vi "rsidr_core_global.vi"() -> ()   [LabVIEW 2020, in "Rohde&Schwarz CMWXP NR FR1 Measurement.lvlib"] (continued)
"Access"=enum."Read Only", "Range Table"="", "Read Callback"="", "Write Callback"="", "Range Callback"="", "Check Callback"="", "Rngtable Callback"="", "Coerce Callback"="", "Supported Models"="", "Instrument Options"="", "Check Status Callback"="", "Flags"=0, "Help"="Returns the values of the power dynamics traces. Each value is sampled with 48 Ts, corresponding to 1.5625 us. The results of the maximum traces can be retrieved.\n\nAvailable Repeated Capabilities:\ninstance: i0, i1, i2, i3, i4, i5, i6, i7, i8, i9, i10, i11, i12, i13, i14, i15, i16, i17, i18, i19, i20, i21, i22, i23, i24, i25, i26, i27, i28, i29, i30, i31, i32\r\n\nRemote-control command(s):\nFETCh:NRSub:MEAS<i>:PRACh:TRACe:PDYNamics:MAXimum?"}, {"Level"=3, "Class Only"=TRUE, "Identifier"="", "Descriptive Name"="Modulation", "Data Type"=enum."ViInt32", "Command"="", "Access"=enum."Read Only", "Range Table"="", "Read Callback"="", "Write Callback"="", "Range Callback"="", "Check Callback"="", "Rngtable Callback"="", "Coerce Callback"="", "Supported Models"="", "Instrument Options"="", "Check Status Callback"="", "Flags"=0, "Help"="The following commands return the statistical modulation results."}, {"Level"=4, "Class Only"=FALSE, "Identifier"="RSCMWXPNRFR1M_ATTR_QUERY_PRACH_MODULATION_CURRENT_LIMIT_CHECK_RESULTS", "Descriptive Name"="Query PRACH Modulation Current Limit Check Results", "Data Type"=enum."RawString", "Command"="CALC:NRS:MEAS{instance}:PRAC:MOD:CURR?", "Access"=enum."Read Only", "Range Table"="", "Read Callback"="", "Write Callback"="", "Range Callback"="", "Check Callback"="", "Rngtable Callback"="", "Coerce Callback"="", "Supported Models"="", "Instrument Options"="", "Check Status Callback"="", "Flags"=0, "Help"="Returns the limit check results for the current single value results.\n\nAvailable Repeated Capabilities:\ninstance: i0, i1, i2, i3, i4, i5, i6, i7, i8, i9, i10, i11, i12, i13, i14, i15, i16, i17, i18, i19, i20, i21, i22, i23, i24, i25, i26, i27, i28, i29, i30, i31, i32\r\n\nRemote-control command(s):\nCALCulate:NRSub:MEAS<i>:PRACh:MODulation:CURRent?"}, {"Level"=4, "Class Only"=FALSE, "Identifier"="RSCMWXPNRFR1M_ATTR_QUERY_PRACH_MODULATION_AVERAGE_LIMIT_CHECK_RESULTS", "Descriptive Name"="Query PRACH Modulation Average Limit Check Results", "Data Type"=enum."RawString", "Command"="CALC:NRS:MEAS{instance}:PRAC:MOD:AVER?", "Access"=enum."Read Only", "Range Table"="", "Read Callback"="", "Write Callback"="", "Range Callback"="", "Check Callback"="", "Rngtable Callback"="", "Coerce Callback"="", "Supported Models"="", "Instrument Options"="", "Check Status Callback"="", "Flags"=0, "Help"="Returns the limit check results for the average single value results.\n\nAvailable Repeated Capabilities:\ninstance: i0, i1, i2, i3, i4, i5, i6, i7, i8, i9, i10, i11, i12, i13, i14, i15, i16, i17, i18, i19, i20, i21, i22, i23, i24, i25, i26, i27, i28, i29, i30, i31, i32\r\n\nRemote-control command(s):\nCALCulate:NRSub:MEAS<i>:PRACh:MODulation:AVERage?"}, {"Level"=4, "Class Only"=FALSE, "Identifier"="RSCMWXPNRFR1M_ATTR_READ_PRACH_MODULATION_CURRENT_RESULTS", "Descriptive Name"="Read PRACH Modulation Current Results", "Data Type"=enum."RawString", "Command"="READ:NRS:MEAS{instance}:PRAC:MOD:CURR?", "Access"=enum."Read Only", "Range Table"="", "Read Callback"="", "Write Callback"="", "Range Callback"="", "Check Callback"="", "Rngtable Callback"="", "Coerce Callback"="", "Supported Models"="", "Instrument Options"="", "Check Status Callback"="", "Flags"=0, "Help"="Starts a new single shot measurement and returns the current single value results.\n\nAvailable Repeated Capabilities:\ninstance: i0, i1, i2, i3, i4, i5, i6, i7, i8, i9, i10, i11, i12, i13, i14, i15, i16, i17, i18, i19, i20, i21, i22, i23, i24, i25, i26, i27, i28, i29, i30, i31, i32\r\n\nRemote-control command(s):\nREAD:NRSub:MEAS<i>:PRACh:MODulation:CURRent?"}, {"Level"=4, "Class Only"=FALSE, "Identifier"="RSCMWXPNRFR1M_ATTR_READ_PRACH_MODULATION_AVERAGE_RESULTS", "Descriptive Name"="Read PRACH Modulation Average Results", "Data Type"=enum."RawString", "Command"="READ:NRS:MEAS{instance}:PRAC:MOD:AVER?", "Access"=enum."Read Only", "Range Table"="", "Read Callback"="", "Write Callback"="", "Range Callback"="", "Check Callback"="", "Rngtable Callback"="", "Coerce Callback"="", "Supported Models"="", "Instrument Options"="", "Check Status Callback"="", "Flags"=0, "Help"="Starts a new single shot measurement and returns the average single value results.\n\nAvailable Repeated Capabilities:\ninstance: i0, i1, i2, i3, i4, i5, i6, i7, i8, i9, i10, i11, i12, i13, i14, i15, i16, i17, i18, i19, i20, i21, i22, i23, i24, i25, i26, i27, i28, i29, i30, i31, i32\r\n\nRemote-control command(s):\nREAD:NRSub:MEAS<i>:PRACh:MODulation:AVERage?"}, {"Level"=4, "Class Only"=FALSE, "Identifier"="RSCMWXPNRFR1M_ATTR_READ_PRACH_MODULATION_STANDARD_DEVIATION_RESULTS", "Descriptive Name"="Read PRACH Modulation Standard Deviation Results", "Data Type"=enum."RawString", "Command"="READ:NRS:MEAS{instance}:PRAC:MOD:SDEV?", "Access"=enum."Read Only", "Range Table"="", "Read Callback"="", "Write Callback"="", "Range Callback"="", "Check Callback"="", "Rngtable Callback"="", "Coerce Callback"="", "Supported Models"="", "Instrument Options"="", "Check Status Callback"="", "Flags"=0, "Help"="Starts a new single shot measurement and returns the standard deviation single value results.\n\nAvailable Repeated Capabilities:\ninstance: i0, i1, i2, i3, i4, i5, i6, i7, i8, i9, i10, i11, i12, i13, i14, i15, i16, i17, i18, i19, i20, i21, i22, i23, i24, i25, i26, i27, i28, i29, i30, i31, i32\r\n\nRemote-control command(s):\nREAD:NRSub:MEAS<i>:PRACh:MODulation:SDEViation?"}, {"Level"=4, "Class Only"=FALSE, "Identifier"="RSCMWXPNRFR1M_ATTR_FETCH_PRACH_MODULATION_CURRENT_RESULTS", "Descriptive Name"="Fetch PRACH Modulation Current Results", "Data Type"=enum."RawString", "Command"="FETC:NRS:MEAS{instance}:PRAC:MOD:CURR?", "Access"=enum."Read Only", "Range Table"="", "Read Callback"="", "Write Callback"="", "Range Callback"="", "Check Callback"="", "Rngtable Callback"="", "Coerce Callback"="", "Supported Models"="", "Instrument Options"="", "Check Status Callback"="", "Flags"=0, "Help"="Returns the current single value results.\n\nAvailable Repeated Capabilities:\ninstance: i0, i1, i2, i3, i4, i5, i6, i7, i8, i9, i10, i11, i12, i13, i14, i15, i16, i17, i18, i19, i20, i21, i22, i23, i24, i25, i26, i27, i28, i29, i30, i31, i32\r\n\nRemote-control command(s):\nFETCh:NRSub:MEAS<i>:PRACh:MODulation:CURRent?"}, {"Level"=4, "Class Only"=FALSE, "Identifier"="RSCMWXPNRFR1M_ATTR_FETCH_PRACH_MODULATION_AVERAGE_RESULTS", "Descriptive Name"="Fetch PRACH Modulation Average Results", "Data Type"=enum."RawString", "Command"="FETC:NRS:MEAS{instance}:PRAC:MOD:AVER?", "Access"=enum."Read Only", "Range Table"="", "Read Callback"="", "Write Callback"="", "Range Callback"="", "Check Callback"="", "Rngtable Callback"="", "Coerce Callback"="", "Supported Models"="", "Instrument Options"="", "Check Status Callback"="", "Flags"=0, "Help"="Returns the average single value results.\n\nAvailable Repeated Capabilities:\ninstance: i0, i1, i2, i3, i4, i5, i6, i7, i8, i9, i10, i11, i12, i13, i14, i15, i16, i17, i18, i19, i20, i21, i22, i23, i24, i25, i26, i27, i28, i29, i30, i31, i32\r\n\nRemote-control command(s):\nFETCh:NRSub:MEAS<i>:PRACh:MODulation:AVERage?"}, {"Level"=4, "Class Only"=FALSE, "Identifier"="RSCMWXPNRFR1M_ATTR_FETCH_PRACH_MODULATION_STANDARD_DEVIATION_RESULTS", "Descriptive Name"="Fetch PRACH Modulation Standard Deviation Results", "Data Type"=enum."RawString", "Command"="FETC:NRS:MEAS{instance}:PRAC:MOD:SDEV?", "Access"=enum."Read Only", "Range Table"="", "Read Callback"="", "Write Callback"="", "Range Callback"="", "Check Callback"="", "Rngtable Callback"="", "Coerce Callback"="", "Supported Models"="", "Instrument Options"="", "Check Status Callback"="", "Flags"=0, "Help"="Returns the standard deviation single value results.\n\nAvailable Repeated Capabilities:\ninstance: i0, i1, i2, i3, i4, i5, i6, i7, i8, i9, i10, i11, i12, i13, i14, i15, i16, i17, i18, i19, i20, i21, i22, i23, i24, i25, i26, i27, i28, i29, i30, i31, i32\r\n\nRemote-control command(s):\nFETCh:NRSub:MEAS<i>:PRACh:MODulation:SDEViation?"}, {"Level"=4, "Class Only"=FALSE, "Identifier"="RSCMWXPNRFR1M_ATTR_QUERY_PRACH_MODULATION_EXTREME_LIMIT_CHECK_RESULTS", "Descriptive Name"="Query PRACH Modulation Extreme Limit Check Results", "Data Type"=enum."RawString", "Command"="CALC:NRS:MEAS{instance}:PRAC:MOD:EXTR?", "Access"=enum."Read Only", "Range Table"="", "Read Callback"="", "Write Callback"="", "Range Callback"="", "Check Callback"="", "Rngtable Callback"="", "Coerce Callback"="", "Supported Models"="", "Instrument Options"="", "Check Status Callback"="", "Flags"=0, "Help"="Returns the limit check results for modulation extreme values.\n\nAvailable Repeated Capabilities:\ninstance: i0, i1, i2, i3, i4, i5, i6, i7, i8, i9, i10, i11, i12, i13, i14, i15, i16, i17, i18, i19, i20, i21, i22, i23, i24, i25, i26, i27, i28, i29, i30, i31, i32\r\n\nRemote-control command(s):\nCALCulate:NRSub:MEAS<i>:PRACh:MODulation:EXTReme?"}, {"Level"=4, "Class Only"=FALSE, "Identifier"="RSCMWXPNRFR1M_ATTR_READ_PRACH_MODULATION_EXTREME_RESULTS", "Descriptive Name"="Read PRACH Modulation Extreme Results", "Data Type"=enum."RawString", "Command"="READ:NRS:MEAS{instance}:PRAC:MOD:EXTR?", "Access"=enum."Read Only", "Range Table"="", "Read Callback"="", "Write Callback"="", "Range Callback"="", "Check Callback"="", "Rngtable Callback"="", "Coerce Callback"="", "Supported Models"="", "Instrument Options"="", "Check Status Callback"="", "Flags"=0, "Help"="Starts a new single shot measurement and returns the extreme single value results.\n\nAvailable Repeated Capabilities:\ninstance: i0, i1, i2, i3, i4, i5, i6, i7, i8, i9, i10, i11, i12, i13, i14, i15, i16, i17, i18, i19, i20, i21, i22, i23, i24, i25, i26, i27, i28, i29, i30, i31, i32\r\n\nRemote-control command(s):\nREAD:NRSub:MEAS<i>:PRACh:MODulation:EXTReme?"}, {"Level"=4, "Class Only"=FALSE, "Identifier"="RSCMWXPNRFR1M_ATTR_FETCH_PRACH_MODULATION_EXTREME_RESULTS", "Descriptive Name"="Fetch PRACH Modulation Extreme Results", "Data Type"=enum."RawString", "Command"="FETC:NRS:MEAS{instance}:PRAC:MOD:EXTR?", "Access"=enum."Read Only", "Range Table"="", "Read Callback"="", "Write Callback"="", "Range Callback"="", "Check Callback"="", "Rngtable Callback"="", "Coerce Callback"="", "Supported Models"="", "Instrument Options"="", "Check Status Callback"="", "Flags"=0, "Help"="Returns the extreme single value results.\n\nAvailable Repeated Capabilities:\ninstance: i0, i1, i2, i3, i4, i5, i6, i7, i8, i9, i10, i11, i12, i13, i14, i15, i16, i17, i18, i19, i20, i21, i22, i23, i24, i25, i26, i27, i28, i29, i30, i31, i32\r\n\nRemote-control command(s):\nFETCh:NRSub:MEAS<i>:PRACh:MODulation:EXTReme?"}, {"Level"=4, "Class Only"=FALSE, "Identifier"="RSCMWXPNRFR1M_ATTR_READ_PRACH_MODULATION_EVM_POWER_VS_PREAMBLE_RESULTS", "Descriptive Name"="Read PRACH Modulation EVM / Power Vs Preamble Results", "Data Type"=enum."RawString", "Command"="READ:NRS:MEAS{instance}:PRAC:MOD:PRE{preamble}?", "Access"=enum."Read Only", "Range Table"="", "Read Callback"="", "Write Callback"="", "Range Callback"="", "Check Callback"="", "Rngtable Callback"="", "Coerce Callback"="", "Supported Models"="", "Instrument Options"="", "Check Status Callback"="", "Flags"=0, "Help"="Starts a new single shot measurement and returns the single value results of the 'EVM vs Preamble' and 'Power vs Preamble' squares, for a selected preamble.\n\nAvailable Repeated Capabilities:\ninstance: i0, i1, i2, i3, i4, i5, i6, i7, i8, i9, i10, i11, i12, i13, i14, i15, i16, i17, i18, i19, i20, i21, i22, i23, i24, i25, i26, i27, i28, i29, i30, i31, i32\r\npreamble: p1\r\n\nRemote-control command(s):\nREAD:NRSub:MEAS<i>:PRACh:MODulation:PREamble<Number>?"}, {"Level"=4, "Class Only"=FALSE, "Identifier"="RSCMWXPNRFR1M_ATTR_FETCH_PRACH_MODULATION_EVM_POWER_VS_PREAMBLE_RESULTS", "Descriptive Name"="Fetch PRACH Modulation EVM / Power Vs Preamble Results", "Data Type"=enum."RawString", "Command"="FETC:NRS:MEAS{instance}:PRAC:MOD:PRE{preamble}?", "Access"=enum."Read Only", "Range Table"="", "Read Callback"="", "Write Callback"="", "Range Callback"="", "Check Callback"="", "Rngtable Callback"="", "Coerce Callback"="", "Supported Models"="", "Instrument Options"="", "Check Status Callback"="", "Flags"=0, "Help"="Returns the single value results of the 'EVM vs Preamble' and 'Power vs Preamble' squares, for a selected preamble.\nSee also 'Squares EVM vs Preamble, Power vs Preamble'.\n\nAvailable Repeated Capabilities:\ninstance: i0, i1, i2, i3, i4, i5, i6, i7, i8, i9, i10, i11, i12, i13, i14, i15, i16, i17, i18, i19, i20, i21, i22, i23, i24, i25, i26, i27, i28, i29, i30, i31, i32\r\npreamble: p1\r\n\nRemote-control command(s):\nFETCh:NRSub:MEAS<i>:PRACh:MODulation:PREamble<Number>?"}, {"Level"=1, "Class Only"=TRUE, "Identifier"="", "Descriptive Name"="Utility", "Data Type"=enum."ViInt32", "Command"="", "Access"=enum."Read Only", "Range Table"="", "Read Callback"="", "Write Callback"="", "Range Callback"="", "Check Callback"="", "Rngtable Callback"="", "Coerce Callback"="", "Supported Models"="", "Instrument Options"="", "Check Status Callback"="", "Flags"=0, "Help"="Put a help here"}, {"Level"=2, "Class Only"=FALSE, "Identifier"="RSCMWXPNRFR1M_ATTR_SYSTEM_VERSION", "Descriptive Name"="System Version", "Data Type"=enum."ViString", "Command"="SYST:VERSion?", "Access"=enum."Read Only", "Range Table"="", "Read Callback"="", "Write Callback"="", "Range Callback"="", "Check Callback"="", "Rngtable Callback"="", "Coerce Callback"="", "Supported Models"="", "Instrument Options"="", "Check Status Callback"="", "Flags"=0, "Help"="Gets system version.\n\nAvailable Repeated Capabilities:\nNone\n\nRemote-control command(s):\nSYSTem:VERSion?"}, {"Level"=2, "Class Only"=FALSE, "Identifier"="RSCMWXPNRFR1M_ATTR_SYSTEM_ERROR", "Descriptive Name"="System Error", "Data Type"=enum."ViString", "Command"="SYST:ERRor?", "Access"=enum."Read Only", "Range Table"="", "Read Callback"="", "Write Callback"="", "Range Callback"="", "Check Callback"="", "Rngtable Callback"="", "Coerce Callback"="", "Supported Models"="", "Instrument Options"="", "Check Status Callback"="", "Flags"=0, "Help"="This attribute queries the earliest entry in the error queue, and deletes it after the readout.\n\nAvailable Repeated Capabilities:\nNone\n\nRemote-control command(s):\nSYSTem:ERRor?"}, {"Level"=2, "Class Only"=FALSE, "Identifier"="RSCMWXPNRFR1M_ATTR_SYSTEM_ALL_ERRORS", "Descriptive Name"="System All Errors", "Data Type"=enum."ViString", "Command"="SYST:ERR:ALL?", "Access"=enum."Read Only", "Range Table"="", "Read Callback"="", "Write Callback"="", "Range Callback"="", "Check Callback"="", "Rngtable Callback"="", "Coerce Callback"="", "Supported Models"="", "Instrument Options"="", "Check Status Callback"="", "Flags"=0, "Help"="Reads all errors from instrument.\n\nAvailable Repeated Capabilities:\nNone\n\nRemote-control command(s):\nSYSTem:ERRor:ALL?"}, {"Level"=2, "Class Only"=FALSE, "Identifier"="RSCMWXPNRFR1M_ATTR_SYSTEM_PRESET", "Descriptive Name"="System Preset", "Data Type"=enum."None", "Command"="SYST:PRES", "Access"=enum."Write Only", "Range Table"="", "Read Callback"="", "Write Callback"="", "Range Callback"="", "Check Callback"="", "Rngtable Callback"="", "Coerce Callback"="", "Supported Models"="", "Instrument Options"="", "Check Status Callback"="", "Flags"=0, "Help"="Resets instrument.\n\nAvailable Repeated Capabilities:\nNone\n\nRemote-control command(s):\nSYSTem:PRESet"}, {"Level"=2, "Class Only"=FALSE, "Identifier"="RSCMWXPNRFR1M_ATTR_PROCESS_ALL_PREVIOUS_COMMANDS", "Descriptive Name"="Process All Previous Commands", "Data Type"=enum."None", "Command"="*WAI", "Access"=enum."Write Only", "Range Table"="", "Read Callback"="", "Write Callback"="", "Range Callback"="", "Check Callback"="", "Rngtable Callback"="", "Coerce Callback"="", "Supported Models"="", "Instrument Options"="", "Check Status Callback"="", "Flags"=0, "Help"="Stops further command processing until all commands sent before *WAI have been executed.\n\nAvailable Repeated Capabilities:\nNone\n\nRemote-control command(s):\n*WAI"}] {"Flags" format="%4b"}
  in  "Supported Models":string[](array[string])=["CMX", "CMP", "CMW"]
  in  "Repeated Capabilities":T2(array[cluster])
  in  "Range Tables":T3(array[cluster])=[{"Name"="rsCmwxpNrFr1M_rngBandwidthPart", "Type"=enum."Discrete", "Entries"=[{"Name"="BWP0", "Discrete or Min"=0.0, "Max"=0.0, "Coerced"=0.0, "Command"="BWP0"}]}, {"Name"="rsCmwxpNrFr1M_rngTxBWOffset", "Type"=enum."Range", "Entries"=[{"Name"="", "Discrete or Min"=0.0, "Max"=9.0, "Coerced"=0.0, "Command"=""}]}, {"Name"="rsCmwxpNrFr1M_rngPDYNOFFPower", "Type"=enum."Range", "Entries"=[{"Name"="", "Discrete or Min"=-256.0, "Max"=256.0, "Coerced"=0.0, "Command"=""}]}, {"Name"="rsCmwxpNrFr1M_rngMeasureSlot", "Type"=enum."Discrete", "Entries"=[{"Name"="0", "Discrete or Min"=0.0, "Max"=0.0, "Coerced"=0.0, "Command"="MS0"}, {"Name"="1", "Discrete or Min"=1.0, "Max"=0.0, "Coerced"=0.0, "Command"="MS1"}, {"Name"="2", "Discrete or Min"=2.0, "Max"=0.0, "Coerced"=0.0, "Command"="MS2"}, {"Name"="3", "Discrete or Min"=3.0, "Max"=0.0, "Coerced"=0.0, "Command"="MS3"}, {"Name"="All", "Discrete or Min"=4.0, "Max"=0.0, "Coerced"=0.0, "Command"="ALL"}]}, {"Name"="rsCmwxpNrFr1M_rngStatCount", "Type"=enum."Range", "Entries"=[{"Name"="", "Discrete or Min"=1.0, "Max"=1000.0, "Coerced"=0.0, "Command"=""}]}, {"Name"="rsCmwxpNrFr1M_rngExtAtt", "Type"=enum."Range", "Entries"=[{"Name"="", "Discrete or Min"=-50.0, "Max"=90.0, "Coerced"=0.0, "Command"=""}]}, {"Name"="rsCmwxpNrFr1M_rngMixerLevelOffset", "Type"=enum."Range", "Entries"=[{"Name"="", "Discrete or Min"=-10.0, "Max"=10.0, "Coerced"=0.0, "Command"=""}]}, {"Name"="rsCmwxpNrFr1M_rngPhysicalCellID", "Type"=enum."Range", "Entries"=[{"Name"="", "Discrete or Min"=0.0, "Max"=1007.0, "Coerced"=0.0, "Command"=""}]}, {"Name"="rsCmwxpNrFr1M_rngTypeAPosition", "Type"=enum."Range", "Entries"=[{"Name"="", "Discrete or Min"=2.0, "Max"=3.0, "Coerced"=0.0, "Command"=""}]}, {"Name"="rsCmwxpNrFr1M_rngTrigThreshold", "Type"=enum."Range", "Entries"=[{"Name"="", "Discrete or Min"=-50.0, "Max"=0.0, "Coerced"=0.0, "Command"=""}]}, {"Name"="rsCmwxpNrFr1M_rngConnector", "Type"=enum."Discrete", "Entries"=[{"Name"="Standalone", "Discrete or Min"=0.0, "Max"=0.0, "Coerced"=0.0, "Command"="STAN"}, {"Name"="Network", "Discrete or Min"=1.0, "Max"=0.0, "Coerced"=0.0, "Command"="NETW"}]}, {"Name"="rsCmwxpNrFr1M_rngBand", "Type"=enum."Range", "Entries"=[{"Name"="", "Discrete or Min"=1.0, "Max"=86.0, "Coerced"=0.0, "Command"=""}]}, {"Name"="rsCmwxpNrFr1M_rngFrequencyOffset", "Type"=enum."Range", "Entries"=[{"Name"="", "Discrete or Min"=-100000.0, "Max"=100000.0, "Coerced"=0.0, "Command"=""}]}, {"Name"="rsCmwxpNrFr1M_rngPeriodicity", "Type"=enum."Discrete", "Entries"=[{"Name"="0.5 ms", "Discrete or Min"=0.0, "Max"=0.0, "Coerced"=0.0, "Command"="MS05"}, {"Name"="1 ms", "Discrete or Min"=1.0, "Max"=0.0, "Coerced"=0.0, "Command"="MS1"}, {"Name"="1.25 ms", "Discrete or Min"=2.0, "Max"=0.0, "Coerced"=0.0, "Command"="MS125"}, {"Name"="2 ms", "Discrete or Min"=3.0, "Max"=0.0, "Coerced"=0.0, "Command"="MS2"}, {"Name"="2.5 ms", "Discrete or Min"=4.0, "Max"=0.0, "Coerced"=0.0, "Command"="MS25"}, {"Name"="3 ms", "Discrete or Min"=5.0, "Max"=0.0, "Coerced"=0.0, "Command"="MS3"}, {"Name"="4 ms", "Discrete or Min"=6.0, "Max"=0.0, "Coerced"=0.0, "Command"="MS4"}, {"Name"="5 ms", "Discrete or Min"=7.0, "Max"=0.0, "Coerced"=0.0, "Command"="MS5"}, {"Name"="10 ms", "Discrete or Min"=8.0, "Max"=0.0, "Coerced"=0.0, "Command"="MS10"}]}, {"Name"="rsCmwxpNrFr1M_rngChannelBandwidth", "Type"=enum."Discrete", "Entries"=[{"Name"="5 MHz", "Discrete or Min"=0.0, "Max"=0.0, "Coerced"=0.0, "Command"="B005"}, {"Name"="10 MHz", "Discrete or Min"=1.0, "Max"=0.0, "Coerced"=0.0, "Command"="B010"}, {"Name"="15 MHz", "Discrete or Min"=2.0, "Max"=0.0, "Coerced"=0.0, "Command"="B015"}, {"Name"="20 MHz", "Discrete or Min"=3.0, "Max"=0.0, "Coerced"=0.0, "Command"="B020"}, {"Name"="25 MHz", "Discrete or Min"=4.0, "Max"=0.0, "Coerced"=0.0, "Command"="B025"}, {"Name"="30 MHz", "Discrete or Min"=5.0, "Max"=0.0, "Coerced"=0.0, "Command"="B030"}, {"Name"="40 MHz", "Discrete or Min"=6.0, "Max"=0.0, "Coerced"=0.0, "Command"="B040"}, {"Name"="50 MHz", "Discrete or Min"=7.0, "Max"=0.0, "Coerced"=0.0, "Command"="B050"}, {"Name"="60 MHz", "Discrete or Min"=8.0, "Max"=0.0, "Coerced"=0.0, "Command"="B060"}, {"Name"="80 MHz", "Discrete or Min"=9.0, "Max"=0.0, "Coerced"=0.0, "Command"="B080"}, {"Name"="90 MHz", "Discrete or Min"=10.0, "Max"=0.0, "Coerced"=0.0, "Command"="B090"}, {"Name"="100 MHz", "Discrete or Min"=11.0, "Max"=0.0, "Coerced"=0.0, "Command"="B100"}]}, {"Name"="rsCmwxpNrFr1M_rngNumberOfRBs", "Type"=enum."Range", "Entries"=[{"Name"="", "Discrete or Min"=11.0, "Max"=273.0, "Coerced"=0.0, "Command"=""}]}, {"Name"="rsCmwxpNrFr1M_rngStartRB", "Type"=enum."Range", "Entries"=[{"Name"="", "Discrete or Min"=0.0, "Max"=262.0, "Coerced"=0.0, "Command"=""}]}, {"Name"="rsCmwxpNrFr1M_rngDMRSConfigType", "Type"=enum."Range", "Entries"=[{"Name"="", "Discrete or Min"=1.0, "Max"=2.0, "Coerced"=0.0, "Command"=""}]}, {"Name"="rsCmwxpNrFr1M_rngDMRSAdditionalPosition", "Type"=enum."Range", "Entries"=[{"Name"="", "Discrete or Min"=0.0, "Max"=3.0, "Coerced"=0.0, "Command"=""}]}, {"Name"="rsCmwxpNrFr1M_rngDMRSMaxLength", "Type"=enum."Range", "Entries"=[{"Name"="", "Discrete or Min"=1.0, "Max"=1.0, "Coerced"=0.0, "Command"=""}]}, {"Name"="rsCmwxpNrFr1M_rngPct", "Type"=enum."Range", "Entries"=[{"Name"="", "Discrete or Min"=0.0, "Max"=100.0, "Coerced"=0.0, "Command"=""}]}, {"Name"="rsCmwxpNrFr1M_rngDeg", "Type"=enum."Range", "Entries"=[{"Name"="", "Discrete or Min"=0.0, "Max"=180.0, "Coerced"=0.0, "Command"=""}]}, {"Name"="rsCmwxpNrFr1M_rngLimitOffset", "Type"=enum."Range", "Entries"=[{"Name"="", "Discrete or Min"=-256.0, "Max"=256.0, "Coerced"=0.0, "Command"=""}]}, {"Name"="rsCmwxpNrFr1M_rngSubcarrierSpacing", "Type"=enum."Discrete", "Entries"=[{"Name"="15 kHz", "Discrete or Min"=0.0, "Max"=0.0, "Coerced"=0.0, "Command"="S15K"}, {"Name"="30 kHz", "Discrete or Min"=1.0, "Max"=0.0, "Coerced"=0.0, "Command"="S30K"}, {"Name"="60 kHz", "Discrete or Min"=2.0, "Max"=0.0, "Coerced"=0.0, "Command"="S60K"}]}, {"Name"="rsCmwxpNrFr1M_rngRepMode", "Type"=enum."Discrete", "Entries"=[{"Name"="Single shot measurement", "Discrete or Min"=0.0, "Max"=0.0, "Coerced"=0.0, "Command"="SING"}, {"Name"="Continuous measurement", "Discrete or Min"=1.0, "Max"=0.0, "Coerced"=0.0, "Command"="CONT"}]}, {"Name"="rsCmwxpNrFr1M_rngStopCondition", "Type"=enum."Discrete", "Entries"=[{"Name"="None", "Discrete or Min"=0.0, "Max"=0.0, "Coerced"=0.0, "Command"="NONE"}, {"Name"="Limit Failure", "Discrete or Min"=1.0, "Max"=0.0, "Coerced"=0.0, "Command"="SLF"}]}, {"Name"="rsCmwxpNrFr1M_rngMeasurementMode", "Type"=enum."Discrete", "Entries"=[{"Name"="Normal", "Discrete or Min"=0.0, "Max"=0.0, "Coerced"=0.0, "Command"="NORM"}, {"Name"="List Mode", "Discrete or Min"=1.0, "Max"=0.0, "Coerced"=0.0, "Command"="MELM"}]}, {"Name"="rsCmwxpNrFr1M_rngMeasFilter", "Type"=enum."Discrete", "Entries"=[{"Name"="Bandpass", "Discrete or Min"=0.0, "Max"=0.0, "Coerced"=0.0, "Command"="BAND"}, {"Name"="Gauss", "Discrete or Min"=1.0, "Max"=0.0, "Coerced"=0.0, "Command"="GAUS"}]}, {"Name"="rsCmwxpNrFr1M_rngTrigSlope", "Type"=enum."Discrete", "Entries"=[{"Name"="Rising", "Discrete or Min"=0.0, "Max"=0.0, "Coerced"=0.0, "Command"="REDG"}, {"Name"="Falling", "Discrete or Min"=1.0, "Max"=0.0, "Coerced"=0.0, "Command"="FEDG"}]}, {"Name"="rsCmwxpNrFr1M_rngMultiEvalMeasurementTriggerDelay", "Type"=enum."Range", "Entries"=[{"Name"="", "Discrete or Min"=-0.00025, "Max"=0.00025, "Coerced"=0.0, "Command"=""}]}, {"Name"="rsCmwxpNrFr1M_rngTriggerTimeout", "Type"=enum."Range", "Entries"=[{"Name"="", "Discrete or Min"=0.01, "Max"=167772.15, "Coerced"=0.0, "Command"=""}]}, {"Name"="rsCmwxpNrFr1M_rngMinimumTriggerGap", "Type"=enum."Range", "Entries"=[{"Name"="", "Discrete or Min"=0.0, "Max"=0.001, "Coerced"=0.0, "Command"=""}]}, {"Name"="rsCmwxpNrFr1M_rngTriggerSyncMode", "Type"=enum."Discrete", "Entries"=[{"Name"="Normal", "Discrete or Min"=0.0, "Max"=0.0, "Coerced"=0.0, "Command"="NORM"}, {"Name"="Enhanced", "Discrete or Min"=1.0, "Max"=0.0, "Coerced"=0.0, "Command"="ENH"}]}, {"Name"="rsCmwxpNrFr1M_rngTriggerListMode", "Type"=enum."Discrete", "Entries"=[{"Name"="Once", "Discrete or Min"=0.0, "Max"=0.0, "Coerced"=0.0, "Command"="ONCE"}, {"Name"="Segment", "Discrete or Min"=1.0, "Max"=0.0, "Coerced"=0.0, "Command"="SEGM"}]}, {"Name"="rsCmwxpNrFr1M_rngLimitOBW", "Type"=enum."Range", "Entries"=[{"Name"="", "Discrete or Min"=0.0, "Max"=120000000.0, "Coerced"=0.0, "Command"=""}]}, {"Name"="rsCmwxpNrFr1M_rngDuplexMode", "Type"=enum."Discrete", "Entries"=[{"Name"="FDD", "Discrete or Min"=0.0, "Max"=0.0, "Coerced"=0.0, "Command"="FDD"}, {"Name"="TDD", "Discrete or Min"=1.0, "Max"=0.0, "Coerced"=0.0, "Command"="TDD"}]}, {"Name"="rsCmwxpNrFr1M_rngNetworkSignaledValue", "Type"=enum."Discrete", "Entries"=[{"Name"="NS01", "Discrete or Min"=1.0, "Max"=0.0, "Coerced"=0.0, "Command"="NS01"}, {"Name"="NS02", "Discrete or Min"=2.0, "Max"=0.0, "Coerced"=0.0, "Command"="NS02"}, {"Name"="NS03", "Discrete or Min"=3.0, "Max"=0.0, "Coerced"=0.0, "Command"="NS03"}, {"Name"="NS04", "Discrete or Min"=4.0, "Max"=0.0, "Coerced"=0.0, "Command"="NS04"}, {"Name"="NS05", "Discrete or Min"=5.0, "Max"=0.0, "Coerced"=0.0, "Command"="NS05"}, {"Name"="NS06", "Discrete or Min"=6.0, "Max"=0.0, "Coerced"=0.0, "Command"="NS06"}, {"Name"="NS07", "Discrete or Min"=7.0, "Max"=0.0, "Coerced"=0.0, "Command"="NS07"}, {"Name"="NS08", "Discrete or Min"=8.0, "Max"=0.0, "Coerced"=0.0, "Command"="NS08"}, {"Name"="NS09", "Discrete or Min"=9.0, "Max"=0.0, "Coerced"=0.0, "Command"="NS09"}, {"Name"="NS10", "Discrete or Min"=10.0, "Max"=0.0, "Coerced"=0.0, "Command"="NS10"}, {"Name"="NS11", "Discrete or Min"=11.0, "Max"=0.0, "Coerced"=0.0, "Command"="NS11"}, {"Name"="NS12", "Discrete or Min"=12.0, "Max"=0.0, "Coerced"=0.0, "Command"="NS12"}, {"Name"="NS13", "Discrete or Min"=13.0, "Max"=0.0, "Coerced"=0.0, "Command"="NS13"}, {"Name"="NS14", "Discrete or Min"=14.0, "Max"=0.0, "Coerced"=0.0, "Command"="NS14"}, {"Name"="NS15", "Discrete or Min"=15.0, "Max"=0.0, "Coerced"=0.0, "Command"="NS15"}, {"Name"="NS16", "Discrete or Min"=16.0, "Max"=0.0, "Coerced"=0.0, "Command"="NS16"}, {"Name"="NS17", "Discrete or Min"=17.0, "Max"=0.0, "Coerced"=0.0, "Command"="NS17"}, {"Name"="NS18", "Discrete or Min"=18.0, "Max"=0.0, "Coerced"=0.0, "Command"="NS18"}, {"Name"="NS19", "Discrete or Min"=19.0, "Max"=0.0, "Coerced"=0.0, "Command"="NS19"}, {"Name"="NS20", "Discrete or Min"=20.0, "Max"=0.0, "Coerced"=0.0, "Command"="NS20"}, {"Name"="NS21", "Discrete or Min"=21.0, "Max"=0.0, "Coerced"=0.0, "Command"="NS21"}, {"Name"="NS22", "Discrete or Min"=22.0, "Max"=0.0, "Coerced"=0.0, "Command"="NS22"}, {"Name"="NS23", "Discrete or Min"=23.0, "Max"=0.0, "Coerced"=0.0, "Command"="NS23"}, {"Name"="NS24", "Discrete or Min"=24.0, "Max"=0.0, "Coerced"=0.0, "Command"="NS24"}, {"Name"="NS25", "Discrete or Min"=25.0, "Max"=0.0, "Coerced"=0.0, "Command"="NS25"}, {"Name"="NS26", "Discrete or Min"=26.0, "Max"=0.0, "Coerced"=0.0, "Command"="NS26"}, {"Name"="NS27", "Discrete or Min"=27.0, "Max"=0.0, "Coerced"=0.0, "Command"="NS27"}, {"Name"="NS28", "Discrete or Min"=28.0, "Max"=0.0, "Coerced"=0.0, "Command"="NS28"}, {"Name"="NS29", "Discrete or Min"=29.0, "Max"=0.0, "Coerced"=0.0, "Command"="NS29"}, {"Name"="NS30", "Discrete or Min"=30.0, "Max"=0.0, "Coerced"=0.0, "Command"="NS30"}, {"Name"="NS31", "Discrete or Min"=31.0, "Max"=0.0, "Coerced"=0.0, "Command"="NS31"}, {"Name"="NS32", "Discrete or Min"=32.0, "Max"=0.0, "Coerced"=0.0, "Command"="NS32"}, {"Name"="NS35", "Discrete or Min"=35.0, "Max"=0.0, "Coerced"=0.0, "Command"="NS35"}]}, {"Name"="rsCmwxpNrFr1M_rngLocation", "Type"=enum."Discrete", "Entries"=[{"Name"="Mid", "Discrete or Min"=0.0, "Max"=0.0, "Coerced"=0.0, "Command"="MID"}, {"Name"="Low", "Discrete or Min"=1.0, "Max"=0.0, "Coerced"=0.0, "Command"="LOW"}, {"Name"="High", "Discrete or Min"=2.0, "Max"=0.0, "Coerced"=0.0, "Command"="HIGH"}, {"Name"="User", "Discrete or Min"=3.0, "Max"=0.0, "Coerced"=0.0, "Command"="USER"}]}, {"Name"="rsCmwxpNrFr1M_rngTDDPeriodicity", "Type"=enum."Discrete", "Entries"=[{"Name"="0.5 ms", "Discrete or Min"=0.0, "Max"=0.0, "Coerced"=0.0, "Command"="P0P5"}, {"Name"="0.6 ms", "Discrete or Min"=1.0, "Max"=0.0, "Coerced"=0.0, "Command"="P0P6"}, {"Name"="1 ms", "Discrete or Min"=2.0, "Max"=0.0, "Coerced"=0.0, "Command"="P1"}, {"Name"="1.2 ms", "Discrete or Min"=3.0, "Max"=0.0, "Coerced"=0.0, "Command"="P1P2"}, {"Name"="2 ms", "Discrete or Min"=4.0, "Max"=0.0, "Coerced"=0.0, "Command"="P2"}, {"Name"="2.5 ms", "Discrete or Min"=5.0, "Max"=0.0, "Coerced"=0.0, "Command"="P2P5"}, {"Name"="3 ms", "Discrete or Min"=6.0, "Max"=0.0, "Coerced"=0.0, "Command"="P3"}, {"Name"="4 ms", "Discrete or Min"=7.0, "Max"=0.0, "Coerced"=0.0, "Command"="P4"}, {"Name"="5 ms", "Discrete or Min"=8.0, "Max"=0.0, "Coerced"=0.0, "Command"="P5"}, {"Name"="10 ms", "Discrete or Min"=9.0, "Max"=0.0, "Coerced"=0.0, "Command"="P10"}]}, {"Name"="rsCmwxpNrFr1M_rngCyclicPrefix", "Type"=enum."Discrete", "Entries"=[{"Name"="Normal", "Discrete or Min"=0.0, "Max"=0.0, "Coerced"=0.0, "Command"="NORM"}, {"Name"="Extended", "Discrete or Min"=1.0, "Max"=0.0, "Coerced"=0.0, "Command"="EXT"}]}, {"Name"="rsCmwxpNrFr1M_rngModulationScheme", "Type"=enum."Discrete", "Entries"=[{"Name"="Auto", "Discrete or Min"=0.0, "Max"=0.0, "Coerced"=0.0, "Command"="AUTO"}, {"Name"="Pi/2-BPSK", "Discrete or Min"=1.0, "Max"=0.0, "Coerced"=0.0, "Command"="BPSK"}, {"Name"="Pi/2-BPSK with shaping", "Discrete or Min"=2.0, "Max"=0.0, "Coerced"=0.0, "Command"="BPWS"}, {"Name"="QPSK", "Discrete or Min"=3.0, "Max"=0.0, "Coerced"=0.0, "Command"="QPSK"}, {"Name"="QAM16", "Discrete or Min"=4.0, "Max"=0.0, "Coerced"=0.0, "Command"="Q16"}, {"Name"="QAM64", "Discrete or Min"=5.0, "Max"=0.0, "Coerced"=0.0, "Command"="Q64"}, {"Name"="QAM256", "Discrete or Min"=6.0, "Max"=0.0, "Coerced"=0.0, "Command"="Q256"}]}, {"Name"="rsCmwxpNrFr1M_rngMappingType", "Type"=enum."Discrete", "Entries"=[{"Name"="A", "Discrete or Min"=0.0, "Max"=0.0, "Coerced"=0.0, "Command"="A"}, {"Name"="B", "Discrete or Min"=1.0, "Max"=0.0, "Coerced"=0.0, "Command"="B"}]}, {"Name"="rsCmwxpNrFr1M_rngDMRSInit", "Type"=enum."Discrete", "Entries"=[{"Name"="Physical Cell ID Used", "Discrete or Min"=0.0, "Max"=0.0, "Coerced"=0.0, "Command"="PHY"}, {"Name"="DMRS ID Used", "Discrete or Min"=1.0, "Max"=0.0, "Coerced"=0.0, "Command"="DID"}]}, {"Name"="rsCmwxpNrFr1M_rngCarrierPosition", "Type"=enum."Discrete", "Entries"=[{"Name"="Left", "Discrete or Min"=0.0, "Max"=0.0, "Coerced"=0.0, "Command"="LONR"}, {"Name"="Right", "Discrete or Min"=1.0, "Max"=0.0, "Coerced"=0.0, "Command"="RONR"}]}, {"Name"="rsCmwxpNrFr1M_rngAreaRBW", "Type"=enum."Discrete", "Entries"=[{"Name"="30 kHz", "Discrete or Min"=0.0, "Max"=0.0, "Coerced"=0.0, "Command"="K030"}, {"Name"="100 kHz", "Discrete or Min"=1.0, "Max"=0.0, "Coerced"=0.0, "Command"="K100"}, {"Name"="1 MHz", "Discrete or Min"=2.0, "Max"=0.0, "Coerced"=0.0, "Command"="M1"}, {"Name"="1 % of channel bandwidth", "Discrete or Min"=3.0, "Max"=0.0, "Coerced"=0.0, "Command"="PC1"}, {"Name"="2 % of channel bandwidth", "Discrete or Min"=4.0, "Max"=0.0, "Coerced"=0.0, "Command"="PC2"}]}, {"Name"="rsCmwxpNrFr1M_rngPhaseCompensation", "Type"=enum."Discrete", "Entries"=[{"Name"="Off", "Discrete or Min"=0.0, "Max"=0.0, "Coerced"=0.0, "Command"="OFF"}, {"Name"="Carrier Frequency", "Discrete or Min"=1.0, "Max"=0.0, "Coerced"=0.0, "Command"="CAF"}, {"Name"="User Defined", "Discrete or Min"=2.0, "Max"=0.0, "Coerced"=0.0, "Command"="UDEF"}]}, {"Name"="rsCmwxpNrFr1M_rngRXConnector", "Type"=enum."Discrete", "Entries"=[{"Name"="RF1C", "Discrete or Min"=0.0, "Max"=0.0, "Coerced"=0.0, "Command"="RF1C"}, {"Name"="RF2C", "Discrete or Min"=1.0, "Max"=0.0, "Coerced"=0.0, "Command"="RF2C"}, {"Name"="RF3C", "Discrete or Min"=2.0, "Max"=0.0, "Coerced"=0.0, "Command"="RF3C"}, {"Name"="RF4C", "Discrete or Min"=3.0, "Max"=0.0, "Coerced"=0.0, "Command"="RF4C"}, {"Name"="R11C", "Discrete or Min"=4.0, "Max"=0.0, "Coerced"=0.0, "Command"="R11C"}, {"Name"="R12C", "Discrete or Min"=5.0, "Max"=0.0, "Coerced"=0.0, "Command"="R12C"}, {"Name"="R13C", "Discrete or Min"=6.0, "Max"=0.0, "Coerced"=0.0, "Command"="R13C"}, {"Name"="R14C", "Discrete or Min"=7.0, "Max"=0.0, "Coerced"=0.0, "Command"="R14C"}, {"Name"="R21C", "Discrete or Min"=8.0, "Max"=0.0, "Coerced"=0.0, "Command"="R21C"}, {"Name"="R22C", "Discrete or Min"=9.0, "Max"=0.0, "Coerced"=0.0, "Command"="R22C"}, {"Name"="R23C", "Discrete or Min"=10.0, "Max"=0.0, "Coerced"=0.0, "Command"="R23C"}, {"Name"="R24C", "Discrete or Min"=11.0, "Max"=0.0, "Coerced"=0.0, "Command"="R24C"}, {"Name"="R31C", "Discrete or Min"=12.0, "Max"=0.0, "Coerced"=0.0, "Command"="R31C"}, {"Name"="R32C", "Discrete or Min"=13.0, "Max"=0.0, "Coerced"=0.0, "Command"="R32C"}, {"Name"="R33C", "Discrete or Min"=14.0, "Max"=0.0, "Coerced"=0.0, "Command"="R33C"}, {"Name"="R34C", "Discrete or Min"=15.0, "Max"=0.0, "Coerced"=0.0, "Command"="R34C"}, {"Name"="R41C", "Discrete or Min"=16.0, "Max"=0.0, "Coerced"=0.0, "Command"="R41C"}, {"Name"="R42C", "Discrete or Min"=17.0, "Max"=0.0, "Coerced"=0.0, "Command"="R42C"}, {"Name"="R43C", "Discrete or Min"=18.0, "Max"=0.0, "Coerced"=0.0, "Command"="R43C"}, {"Name"="R44C", "Discrete or Min"=19.0, "Max"=0.0, "Coerced"=0.0, "Command"="R44C"}]}, {"Name"="rsCmwxpNrFr1M_rngRFConverter", "Type"=enum."Discrete", "Entries"=[{"Name"="RX1", "Discrete or Min"=0.0, "Max"=0.0, "Coerced"=0.0, "Command"="RX1"}, {"Name"="RX2", "Discrete or Min"=1.0, "Max"=0.0, "Coerced"=0.0, "Command"="RX2"}, {"Name"="RX3", "Discrete or Min"=2.0, "Max"=0.0, "Coerced"=0.0, "Command"="RX3"}, {"Name"="RX4", "Discrete or Min"=3.0, "Max"=0.0, "Coerced"=0.0, "Command"="RX4"}, {"Name"="RX11", "Discrete or Min"=4.0, "Max"=0.0, "Coerced"=0.0, "Command"="RX11"}, {"Name"="RX12", "Discrete or Min"=5.0, "Max"=0.0, "Coerced"=0.0, "Command"="RX12"}, {"Name"="RX13", "Discrete or Min"=6.0, "Max"=0.0, "Coerced"=0.0, "Command"="RX13"}, {"Name"="RX14", "Discrete or Min"=7.0, "Max"=0.0, "Coerced"=0.0, "Command"="RX14"}, {"Name"="RX21", "Discrete or Min"=8.0, "Max"=0.0, "Coerced"=0.0, "Command"="RX21"}, {"Name"="RX22", "Discrete or Min"=9.0, "Max"=0.0, "Coerced"=0.0, "Command"="RX22"}, {"Name"="RX23", "Discrete or Min"=10.0, "Max"=0.0, "Coerced"=0.0, "Command"="RX23"}, {"Name"="RX24", "Discrete or Min"=11.0, "Max"=0.0, "Coerced"=0.0, "Command"="RX24"}, {"Name"="RX31", "Discrete or Min"=12.0, "Max"=0.0, "Coerced"=0.0, "Command"="RX31"}, {"Name"="RX32", "Discrete or Min"=13.0, "Max"=0.0, "Coerced"=0.0, "Command"="RX32"}, {"Name"="RX33", "Discrete or Min"=14.0, "Max"=0.0, "Coerced"=0.0, "Command"="RX33"}, {"Name"="RX34", "Discrete or Min"=15.0, "Max"=0.0, "Coerced"=0.0, "Command"="RX34"}, {"Name"="RX41", "Discrete or Min"=16.0, "Max"=0.0, "Coerced"=0.0, "Command"="RX41"}, {"Name"="RX42", "Discrete or Min"=17.0, "Max"=0.0, "Coerced"=0.0, "Command"="RX42"}, {"Name"="RX43", "Discrete or Min"=18.0, "Max"=0.0, "Coerced"=0.0, "Command"="RX43"}, {"Name"="RX44", "Discrete or Min"=19.0, "Max"=0.0, "Coerced"=0.0, "Command"="RX44"}]}, {"Name"="rsCmwxpNrFr1M_rngRelativeLevel", "Type"=enum."Range", "Entries"=[{"Name"="", "Discrete or Min"=-256.0, "Max"=256.0, "Coerced"=0.0, "Command"=""}]}, {"Name"="rsCmwxpNrFr1M_rngFERR", "Type"=enum."Range", "Entries"=[{"Name"="", "Discrete or Min"=0.0, "Max"=1.0, "Coerced"=0.0, "Command"=""}]}, {"Name"="rsCmwxpNrFr1M_rngResultType", "Type"=enum."Discrete", "Entries"=[{"Name"="Current", "Discrete or Min"=0.0, "Max"=0.0, "Coerced"=0.0, "Command"="CURRENT"}, {"Name"="Average", "Discrete or Min"=1.0, "Max"=0.0, "Coerced"=0.0, "Command"="AVERAGE"}, {"Name"="Extreme", "Discrete or Min"=2.0, "Max"=0.0, "Coerced"=0.0, "Command"="EXTREME"}, {"Name"="Standard Deviation", "Discrete or Min"=3.0, "Max"=0.0, "Coerced"=0.0, "Command"="STANDARD_DEVIATION"}, {"Name"="Maximum", "Discrete or Min"=4.0, "Max"=0.0, "Coerced"=0.0, "Command"="MAXIMUM"}, {"Name"="Minimum", "Discrete or Min"=5.0, "Max"=0.0, "Coerced"=0.0, "Command"="MINIMUM"}]}, {"Name"="rsCmwxpNrFr1M_rngWindowPosition", "Type"=enum."Discrete", "Entries"=[{"Name"="Low", "Discrete or Min"=0.0, "Max"=0.0, "Coerced"=0.0, "Command"="LOW"}, {"Name"="High", "Discrete or Min"=1.0, "Max"=0.0, "Coerced"=0.0, "Command"="HIGH"}]}, {"Name"="rsCmwxpNrFr1M_rngNegPos", "Type"=enum."Discrete", "Entries"=[{"Name"="Negative", "Discrete or Min"=0.0, "Max"=0.0, "Coerced"=0.0, "Command"="NEGATIVE"}, {"Name"="Positive", "Discrete or Min"=1.0, "Max"=0.0, "Coerced"=0.0, "Command"="POSITIVE"}]}, {"Name"="rsCmwxpNrFr1M_rngMinMax", "Type"=enum."Discrete", "Entries"=[{"Name"="Minimum", "Discrete or Min"=0.0, "Max"=0.0, "Coerced"=0.0, "Command"="MIN"}, {"Name"="Maximum", "Discrete or Min"=1.0, "Max"=0.0, "Coerced"=0.0, "Command"="MAX"}]}, {"Name"="rsCmwxpNrFr1M_rngLimitCheckResults", "Type"=enum."Discrete", "Entries"=[{"Name"="Pass", "Discrete or Min"=0.0, "Max"=0.0, "Coerced"=0.0, "Command"="OK"}, {"Name"="Failed Upper", "Discrete or Min"=1.0, "Max"=0.0, "Coerced"=0.0, "Command"="ULEU"}, {"Name"="Failed Lower", "Discrete or Min"=2.0, "Max"=0.0, "Coerced"=0.0, "Command"="ULEL"}, {"Name"="Overflow", "Discrete or Min"=3.0, "Max"=0.0, "Coerced"=0.0, "Command"="OFL"}, {"Name"="Underflow", "Discrete or Min"=4.0, "Max"=0.0, "Coerced"=0.0, "Command"="UFL"}, {"Name"="Invalid", "Discrete or Min"=5.0, "Max"=0.0, "Coerced"=0.0, "Command"="INV"}, {"Name"="Not A Value", "Discrete or Min"=6.0, "Max"=0.0, "Coerced"=0.0, "Command"="NAV"}, {"Name"="Off", "Discrete or Min"=7.0, "Max"=0.0, "Coerced"=0.0, "Command"="OFF"}, {"Name"="Not Capable", "Discrete or Min"=8.0, "Max"=0.0, "Coerced"=0.0, "Command"="NCAP"}]}, {"Name"="rsCmwxpNrFr1M_rngMultiEvalMeasRBW", "Type"=enum."Discrete", "Entries"=[{"Name"="30 kHz", "Discrete or Min"=0.0, "Max"=0.0, "Coerced"=0.0, "Command"="K030"}, {"Name"="100 kHz", "Discrete or Min"=1.0, "Max"=0.0, "Coerced"=0.0, "Command"="K100"}, {"Name"="1 MHz", "Discrete or Min"=2.0, "Max"=0.0, "Coerced"=0.0, "Command"="M1"}, {"Name"="1% of channel BW", "Discrete or Min"=3.0, "Max"=0.0, "Coerced"=0.0, "Command"="PC1"}, {"Name"="2% of channel BW", "Discrete or Min"=4.0, "Max"=0.0, "Coerced"=0.0, "Command"="PC2"}]}, {"Name"="rsCmwxpNrFr1M_rngModScheme", "Type"=enum."Discrete", "Entries"=[{"Name"="Not a value", "Discrete or Min"=-1.0, "Max"=0.0, "Coerced"=0.0, "Command"="NAV"}, {"Name"="Pi/2-BPSK", "Discrete or Min"=0.0, "Max"=0.0, "Coerced"=0.0, "Command"="BPSK"}, {"Name"="Pi/2-BPSK with shaping", "Discrete or Min"=1.0, "Max"=0.0, "Coerced"=0.0, "Command"="BPWS"}, {"Name"="QPSK", "Discrete or Min"=2.0, "Max"=0.0, "Coerced"=0.0, "Command"="QPSK"}, {"Name"="16-QAM", "Discrete or Min"=3.0, "Max"=0.0, "Coerced"=0.0, "Command"="Q16"}, {"Name"="64-QAM", "Discrete or Min"=4.0, "Max"=0.0, "Coerced"=0.0, "Command"="Q64"}, {"Name"="256-QAM", "Discrete or Min"=5.0, "Max"=0.0, "Coerced"=0.0, "Command"="Q256"}]}, {"Name"="rsCmwxpNrFr1M_rngMeasurementMainState", "Type"=enum."Discrete", "Entries"=[{"Name"="Off", "Discrete or Min"=0.0, "Max"=0.0, "Coerced"=0.0, "Command"="OFF"}, {"Name"="Running", "Discrete or Min"=1.0, "Max"=0.0, "Coerced"=0.0, "Command"="RUN"}, {"Name"="Ready", "Discrete or Min"=2.0, "Max"=0.0, "Coerced"=0.0, "Command"="RDY"}]}, {"Name"="rsCmwxpNrFr1M_rngtMeasurementSyncState", "Type"=enum."Discrete", "Entries"=[{"Name"="Pending", "Discrete or Min"=0.0, "Max"=0.0, "Coerced"=0.0, "Command"="PEND"}, {"Name"="Adjusted", "Discrete or Min"=1.0, "Max"=0.0, "Coerced"=0.0, "Command"="ADJ"}, {"Name"="Invalid", "Discrete or Min"=2.0, "Max"=0.0, "Coerced"=0.0, "Command"="INV"}]}, {"Name"="rsCmwxpNrFr1M_rngMeasurementResourceState", "Type"=enum."Discrete", "Entries"=[{"Name"="Queued", "Discrete or Min"=0.0, "Max"=0.0, "Coerced"=0.0, "Command"="QUE"}, {"Name"="Active", "Discrete or Min"=1.0, "Max"=0.0, "Coerced"=0.0, "Command"="ACT"}, {"Name"="Invalid", "Discrete or Min"=2.0, "Max"=0.0, "Coerced"=0.0, "Command"="INV"}]}, {"Name"="rsCmwxpNrFr1M_rngRFUpconversion", "Type"=enum."Range", "Entries"=[{"Name"="", "Discrete or Min"=0.0, "Max"=0.0, "Coerced"=0.0, "Command"=""}]}, {"Name"="rsCmwxpNrFr1M_rngRetriggerFlag", "Type"=enum."Discrete", "Entries"=[{"Name"="Off", "Discrete or Min"=0.0, "Max"=0.0, "Coerced"=0.0, "Command"="OFF"}, {"Name"="On", "Discrete or Min"=1.0, "Max"=0.0, "Coerced"=0.0, "Command"="ON"}, {"Name"="IF Power", "Discrete or Min"=2.0, "Max"=0.0, "Coerced"=0.0, "Command"="IFP"}]}, {"Name"="rsCmwxpNrFr1M_rngPRACHRepetition", "Type"=enum."Discrete", "Entries"=[{"Name"="Single shot measurement", "Discrete or Min"=0.0, "Max"=0.0, "Coerced"=0.0, "Command"="SING"}, {"Name"="Continuous measurement", "Discrete or Min"=1.0, "Max"=0.0, "Coerced"=0.0, "Command"="CONT"}]}, {"Name"="rsCmwxpNrFr1M_rngPRACHStopCondition", "Type"=enum."Discrete", "Entries"=[{"Name"="None", "Discrete or Min"=0.0, "Max"=0.0, "Coerced"=0.0, "Command"="NONE"}, {"Name"="Limit Failure", "Discrete or Min"=1.0, "Max"=0.0, "Coerced"=0.0, "Command"="SLF"}]}, {"Name"="rsCmwxpNrFr1M_rngPRACHNumberOfPreambles", "Type"=enum."Range", "Entries"=[{"Name"="", "Discrete or Min"=1.0, "Max"=1.0, "Coerced"=0.0, "Command"=""}]}, {"Name"="rsCmwxpNrFr1M_rngPRACHStatisticCount", "Type"=enum."Range", "Entries"=[{"Name"="", "Discrete or Min"=1.0, "Max"=1000.0, "Coerced"=0.0, "Command"=""}]}, {"Name"="rsCmwxpNrFr1M_rngPRACHEVMWindowPosition", "Type"=enum."Discrete", "Entries"=[{"Name"="Low", "Discrete or Min"=0.0, "Max"=0.0, "Coerced"=0.0, "Command"="LOW"}, {"Name"="High", "Discrete or Min"=1.0, "Max"=0.0, "Coerced"=0.0, "Command"="HIGH"}]}, {"Name"="rsCmwxpNrFr1M_rngPRACHPowerStatisticCount", "Type"=enum."Range", "Entries"=[{"Name"="", "Discrete or Min"=1.0, "Max"=1000.0, "Coerced"=0.0, "Command"=""}]}, {"Name"="rsCmwxpNrFr1M_rngPRACHTriggerSlope", "Type"=enum."Discrete", "Entries"=[{"Name"="Rising edge", "Discrete or Min"=0.0, "Max"=0.0, "Coerced"=0.0, "Command"="REDG"}, {"Name"="Falling edge", "Discrete or Min"=1.0, "Max"=0.0, "Coerced"=0.0, "Command"="FEDG"}]}, {"Name"="rsCmwxpNrFr1M_rngPRACHTriggerThreshold", "Type"=enum."Range", "Entries"=[{"Name"="", "Discrete or Min"=-50.0, "Max"=0.0, "Coerced"=0.0, "Command"=""}]}, {"Name"="rsCmwxpNrFr1M_rngPRACHTriggerTimeout", "Type"=enum."Range", "Entries"=[{"Name"="", "Discrete or Min"=0.01, "Max"=167772.15, "Coerced"=0.0, "Command"=""}]}, {"Name"="rsCmwxpNrFr1M_rngPRACHMinimumTriggerGap", "Type"=enum."Range", "Entries"=[{"Name"="", "Discrete or Min"=0.0, "Max"=0.001, "Coerced"=0.0, "Command"=""}]}, {"Name"="rsCmwxpNrFr1M_rngPRACHLimitFrequencyError", "Type"=enum."Range", "Entries"=[{"Name"="", "Discrete or Min"=0.0, "Max"=1000.0, "Coerced"=0.0, "Command"=""}]}, {"Name"="rsCmwxpNrFr1M_rngPRACHConfigurationIndex", "Type"=enum."Range", "Entries"=[{"Name"="", "Discrete or Min"=0.0, "Max"=255.0, "Coerced"=0.0, "Command"=""}]}, {"Name"="rsCmwxpNrFr1M_rngPRACHSubcarrierSpacing", "Type"=enum."Discrete", "Entries"=[{"Name"="1.25 kHz", "Discrete or Min"=0.0, "Max"=0.0, "Coerced"=0.0, "Command"="S1K2"}, {"Name"="5 kHz", "Discrete or Min"=1.0, "Max"=0.0, "Coerced"=0.0, "Command"="S5K"}, {"Name"="15 kHz", "Discrete or Min"=2.0, "Max"=0.0, "Coerced"=0.0, "Command"="S15K"}, {"Name"="30 kHz", "Discrete or Min"=3.0, "Max"=0.0, "Coerced"=0.0, "Command"="S30K"}, {"Name"="60 kHz", "Discrete or Min"=4.0, "Max"=0.0, "Coerced"=0.0, "Command"="S60K"}]}, {"Name"="rsCmwxpNrFr1M_rngPRACHLogicalRootSequence", "Type"=enum."Range", "Entries"=[{"Name"="", "Discrete or Min"=0.0, "Max"=837.0, "Coerced"=0.0, "Command"=""}]}, {"Name"="rsCmwxpNrFr1M_rngPRACHZeroCorrelationZone", "Type"=enum."Range", "Entries"=[{"Name"="", "Discrete or Min"=0.0, "Max"=15.0, "Coerced"=0.0, "Command"=""}]}, {"Name"="rsCmwxpNrFr1M_rngPRACHSequenceIndex", "Type"=enum."Range", "Entries"=[{"Name"="", "Discrete or Min"=0.0, "Max"=63.0, "Coerced"=0.0, "Command"=""}]}, {"Name"="rsCmwxpNrFr1M_rngNoSymbols", "Type"=enum."Range", "Entries"=[{"Name"="", "Discrete or Min"=4.0, "Max"=14.0, "Coerced"=0.0, "Command"=""}]}, {"Name"="rsCmwxpNrFr1M_rngStartSymbol", "Type"=enum."Range", "Entries"=[{"Name"="", "Discrete or Min"=0.0, "Max"=10.0, "Coerced"=0.0, "Command"=""}]}, {"Name"="rsCmwxpNrFr1M_rngNoRBs", "Type"=enum."Range", "Entries"=[{"Name"="", "Discrete or Min"=1.0, "Max"=273.0, "Coerced"=0.0, "Command"=""}]}, {"Name"="rsCmwxpNrFr1M_rngStartRBAlloc", "Type"=enum."Range", "Entries"=[{"Name"="", "Discrete or Min"=0.0, "Max"=273.0, "Coerced"=0.0, "Command"=""}]}, {"Name"="rsCmwxpNrFr1M_rngTolerance", "Type"=enum."Range", "Entries"=[{"Name"="", "Discrete or Min"=-3.0, "Max"=3.0, "Coerced"=0.0, "Command"=""}]}, {"Name"="rsCmwxpNrFr1M_rngStartIndex", "Type"=enum."Range", "Entries"=[{"Name"="", "Discrete or Min"=1.0, "Max"=2000.0, "Coerced"=0.0, "Command"=""}]}, {"Name"="rsCmwxpNrFr1M_rngEVMSymbol", "Type"=enum."Range", "Entries"=[{"Name"="", "Discrete or Min"=0.0, "Max"=13.0, "Coerced"=0.0, "Command"=""}]}, {"Name"="rsCmwxpNrFr1M_rngFreqStartEnd", "Type"=enum."Range", "Entries"=[{"Name"="", "Discrete or Min"=0.0, "Max"=405000000.0, "Coerced"=0.0, "Command"=""}]}, {"Name"="rsCmwxpNrFr1M_rngDMRSID", "Type"=enum."Range", "Entries"=[{"Name"="", "Discrete or Min"=0.0, "Max"=65535.0, "Coerced"=0.0, "Command"=""}]}, {"Name"="rsCmwxpNrFr1M_rngnSCID", "Type"=enum."Range", "Entries"=[{"Name"="", "Discrete or Min"=0.0, "Max"=1.0, "Coerced"=0.0, "Command"=""}]}, {"Name"="rsCmwxpNrFr1M_rngEvaluationOffset", "Type"=enum."Range", "Entries"=[{"Name"="", "Discrete or Min"=0.0, "Max"=1000.0, "Coerced"=0.0, "Command"=""}]}, {"Name"="rsCmwxpNrFr1M_rngPctDBL", "Type"=enum."Range", "Entries"=[{"Name"="", "Discrete or Min"=0.0, "Max"=100.0, "Coerced"=0.0, "Command"=""}]}, {"Name"="rsCmwxpNrFr1M_rngEdgeFrequency", "Type"=enum."Range", "Entries"=[{"Name"="", "Discrete or Min"=0.0, "Max"=20000000.0, "Coerced"=0.0, "Command"=""}]}]
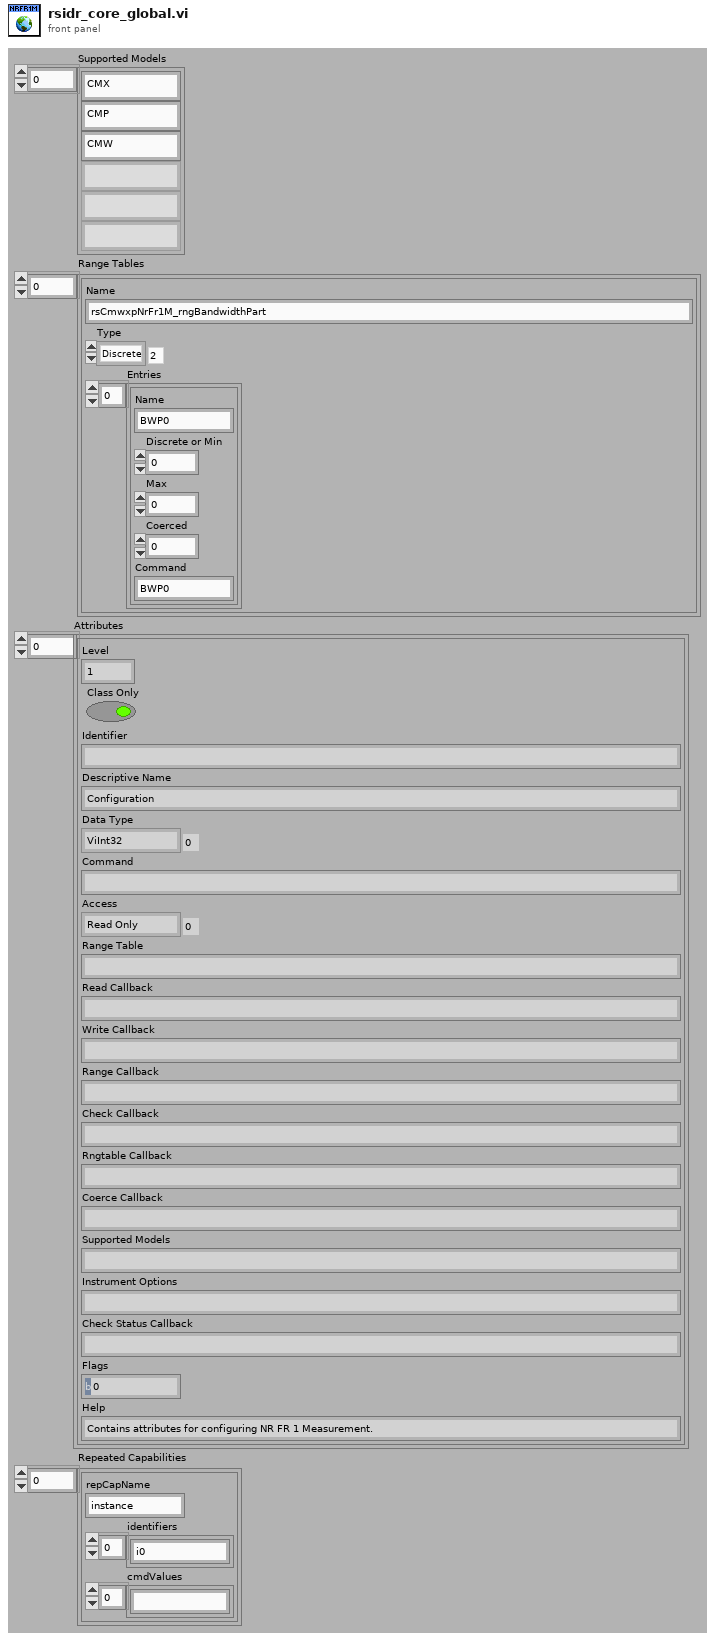
[diagram p1: front panel]
types:
  T1 = cluster{"Level":i32, "Class Only":bool, "Identifier":string, "Descriptive Name":string, "Data Type":enum16{"ViInt32", "ViReal64", "ViString", "ViBoolean", "None", "ViInt64", "RawString"}, "Command":string, "Access":enum16{"Read Only", "Write Only", "Read/Write"}, "Range Table":string, "Read Callback":string, "Write Callback":string, "Range Callback":string, "Check Callback":string, "Rngtable Callback":string, "Coerce Callback":string, "Supported Models":string, "Instrument Options":string, "Check Status Callback":string, "Flags":i32, "Help":string}[]
  T2 = cluster{"repCapName":string, "identifiers":string[], "cmdValues":string[]}[]
  T3 = cluster{"Name":string, "Type":enum16{"Range", "Coerced", "Discrete"}, "Entries":cluster{"Name":string, "Discrete or Min":dbl, "Max":dbl, "Coerced":dbl, "Command":string}[]}[]
diagram:
